vi "Main - Parse Data Tab (SubVI).vi"(11 "NewVal":T2) -> (0 "Bg":bool[](array[boolean]), 1 "Ok":bool[](array[boolean]), 2 "Cancel":bool[](array[boolean]), 3 "Tab":T1(array[cluster]), 4 "Run Test":refnum<vi>[](array[refnum]))   [LabVIEW 2019]
uses:
  Controls/Tab Button.ctl
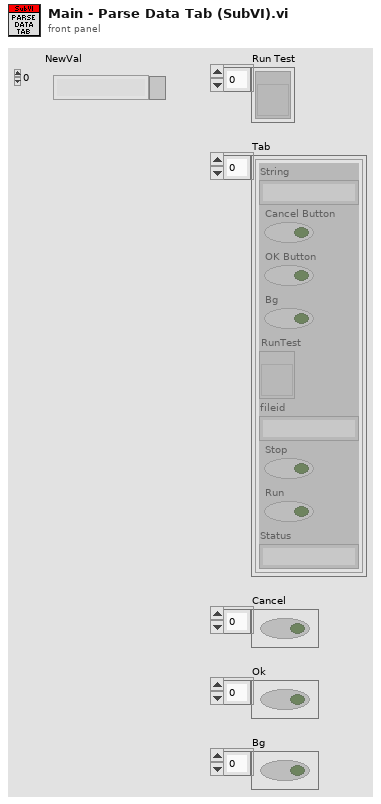
[diagram p1: front panel]
types:
  T1 = cluster{"String":string, "Cancel Button":bool, "OK Button":bool, "Bg":bool, "RunTest":refnum<vi>, "fileid":string, "Stop":bool, "Run":bool, "Status":string}[]
  T2 = typedef "Tab Button.ctl" = cluster{"String":string, "Cancel Button":bool, "OK Button":bool, "Bg":bool, "RunTest":refnum<vi>, "fileid":string, "Stop":bool, "Run":bool, "Status":string}[]
  T3 = cluster{"String":string, "Cancel Button":bool, "OK Button":bool, "Bg":bool, "RunTest":refnum<vi>, "fileid":string, "Stop":bool, "Run":bool, "Status":string}
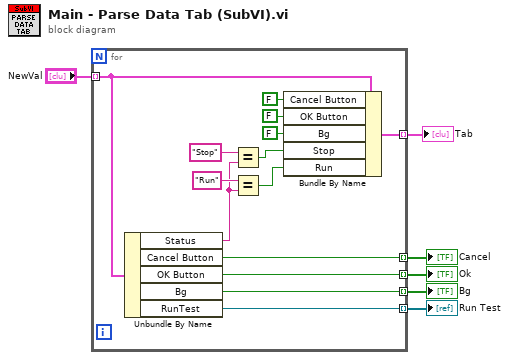
[diagram p0: block diagram]
diagram:
  n1 = for {
    tunnel: "NewVal" -> [w18] mode=indexing
    tunnel: [w20] -> w4 mode=indexing
    tunnel: [w19] -> w3 mode=indexing
    tunnel: [w15] -> w2 mode=indexing
    tunnel: [w13] -> w1 mode=indexing
    tunnel: [w12] -> w6 mode=indexing
    n2 = Unbundle By Name(w18) -> ("Status"=w9:string, "Cancel Button"=w20:bool, "OK Button"=w19:bool, "Bg"=w13:bool, "RunTest"=w12:refnum<vi>)
    n3 = Equal?(x="Stop", y=w9) -> (x = y?=w8:bool)
    n4 = Equal?(x="Run", y=w9) -> (x = y?=w7:bool)
    n5 = Bundle By Name(cluster=w18, "Cancel Button"=FALSE, "OK Button"=FALSE, "Bg"=FALSE, "Stop"=w8, "Run"=w7) -> (w15:T3)
  }
  "Run Test" <- w6
  "Cancel" <- w4
  "Ok" <- w3
  "Tab" <- w2
  "Bg" <- w1
